vi "MultiChannelFeedbackCooling(Host).vi"(5 "RIO Device":T2="RIO0::INSTR") -> ()   [LabVIEW 2012]
doc: "This VI will will initialize the FPGA VI and then continually read and convert single point values from 4 channels of an analog input module."
uses:
  <vilib>/userdefined/High Color/nirio_resource_hc.ctl
  <vilib>/rvi/Analysis/host/Butterworth/config/Butterworth Filter Order.ctl
  <vilib>/rvi/Analysis/host/Butterworth/config/Butterworth Filter Type.ctl
  <vilib>/FPGAPlugInAG/PCIe-7841R/niLvFpga_Open_PCIe-7841R.vi
  <vilib>/FPGAPlugInAG/PCIe-7841R/niLvFpga_Run_PCIe-7841R.vi
  <vilib>/rvi/Analysis/host/Butterworth/config/BwScaledCoefficients.vi
  <vilib>/Utility/error.llb/Error Cluster From Error Code.vi
  <vilib>/rvi/errors/niLvFpgaAdjustHostInterfaceError.vi
  <vilib>/FPGAPlugInAG/PCIe-7841R/niLvFpga_Close_PCIe-7841R.vi
  <vilib>/rvi/interface/nirviOpenFPGA/nirviOpenFPGA.xnode
  MultiChannelFeed_FPGATarget2_feedbackcooling(_T5hmXv3JUos.lvbitx
  <vilib>/rvi/interface/nirviMethod/nirviMethod.xnode
  <vilib>/rvi/Analysis/host/Butterworth/XNode/ButterworthCoefficients.xnode
  <vilib>/rvi/interface/nirviReadWriteControl/nirviReadWriteControl.xnode
  <vilib>/rvi/interface/nirviCloseFPGA/nirviCloseFPGA.xnode
  <vilib>/rvi/Analysis/host/Public/NI_FpgaMspHost.lvlib
  NiFpgaLv.dll
panel:
  in  "feedback gain":fxp<+/-,32,16>
  in  "On time (s)":dbl
  in  "Off time (s)":dbl
  in  "Num cycles":u16
  in  "cycle feedback":bool
  in  "Reset after samps":u16
  in  "Num samps to reset":u16
  in  "change pars 2":bool
  in  "Delay Time (s)":dbl
  in  "Step":fxp<+/-,32,16>
  in  "End value":fxp<+/-,32,16>
  in  "ramp dc offset":bool
  in  "3, 1":fxp<+/-,32,16>
  in  "3, 2":fxp<+/-,32,16>
  in  "3, 3":fxp<+/-,32,16>=1.0
  in  "2, 3":fxp<+/-,32,16>
  in  "2, 2":fxp<+/-,32,16>=1.0
  in  "2, 1":fxp<+/-,32,16>
  in  "1, 3":fxp<+/-,32,16>
  in  "1, 2":fxp<+/-,32,16>
  in  "1,1":fxp<+/-,32,16>=1.0
  out "Feedback 2":dbl(graph)
  out "Filtered Input 2":dbl(graph)=3346.0
  out "AI2":i16(graph)=3346
  out "Feedback 1":dbl(graph)
  out "Filtered Input 1":dbl(graph)=-106.0
  out "AI1":i16(graph)=-104
  out "Feedback 0":dbl(graph)=20.0
  out "Filtered Input 0":dbl(graph)=-40.0
  out "AI0":i16(graph)=-41
  in  "Der delay 2":T1(ring)=enum."4"
  in  "Dc offset 2":fxp<+/-,32,16>
  in  "Lower lim 2":fxp<+/-,32,16>=-1000.0
  in  "Upper lim 2":fxp<+/-,32,16>=1000.0
  in  "dg 2":fxp<+/-,32,16>
  in  "pg 2":fxp<+/-,32,16>
  in  "Setpoint 2":fxp<+/-,16,16>
  in  "Der delay 1":T1(ring)=enum."4"
  in  "cutoff 1 (Hz)":dbl=50000.0
  in  "Dc offset 1":fxp<+/-,32,16>
  in  "Upper lim 1":fxp<+/-,32,16>=3600.0
  in  "Lower lim 1":fxp<+/-,32,16>=-3600.0
  in  "dg 1":fxp<+/-,32,16>
  in  "pg 1":fxp<+/-,32,16>
  in  "Setpoint 1":fxp<+/-,16,16>
  in  "sample rate (S/s)":dbl=120000.0
  in  "cutoff 0 (Hz)":dbl=50000.0
  in  "Der delay 0":T1(ring)=enum."4"
  in  "Dc offset 0":fxp<+/-,32,16>
  in  "Lower lim 0":fxp<+/-,32,16>=-3600.0
  in  "Upper lim 0":fxp<+/-,32,16>=3600.0
  in  "dg 0":fxp<+/-,32,16>=-20.0
  in  "pg 0":fxp<+/-,32,16>
  in  "Setpoint 0":fxp<+/-,16,16>
  in  "change pars":bool
  in  "stop":bool
  # "Analog Input"
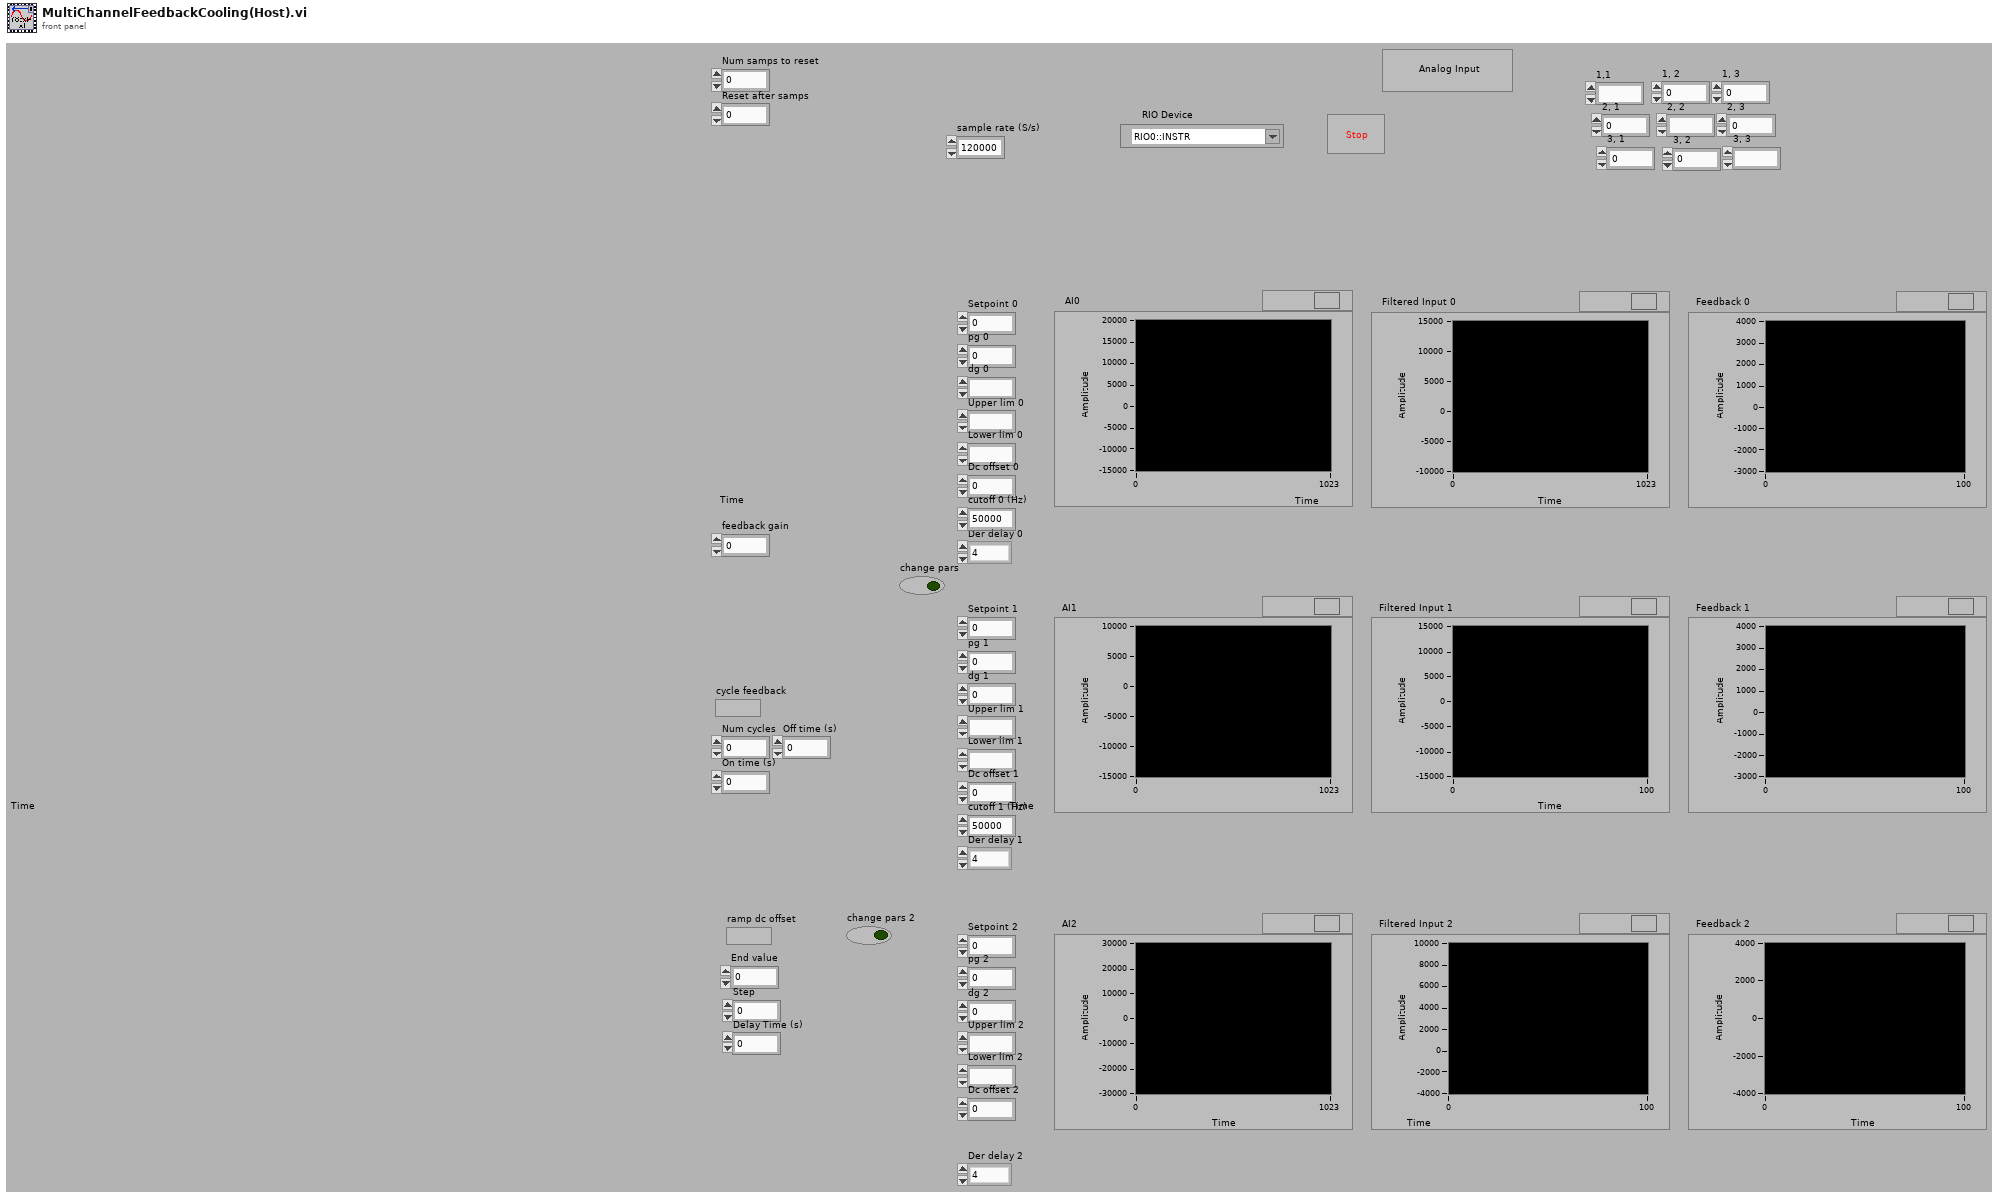
[diagram p1: front panel]
types:
  T1 = enum16{"1", "2", "4", "8", "16", "32", "64", "128", "256", "512"}
  T2 = typedef "nirio_resource_hc.ctl" = tag
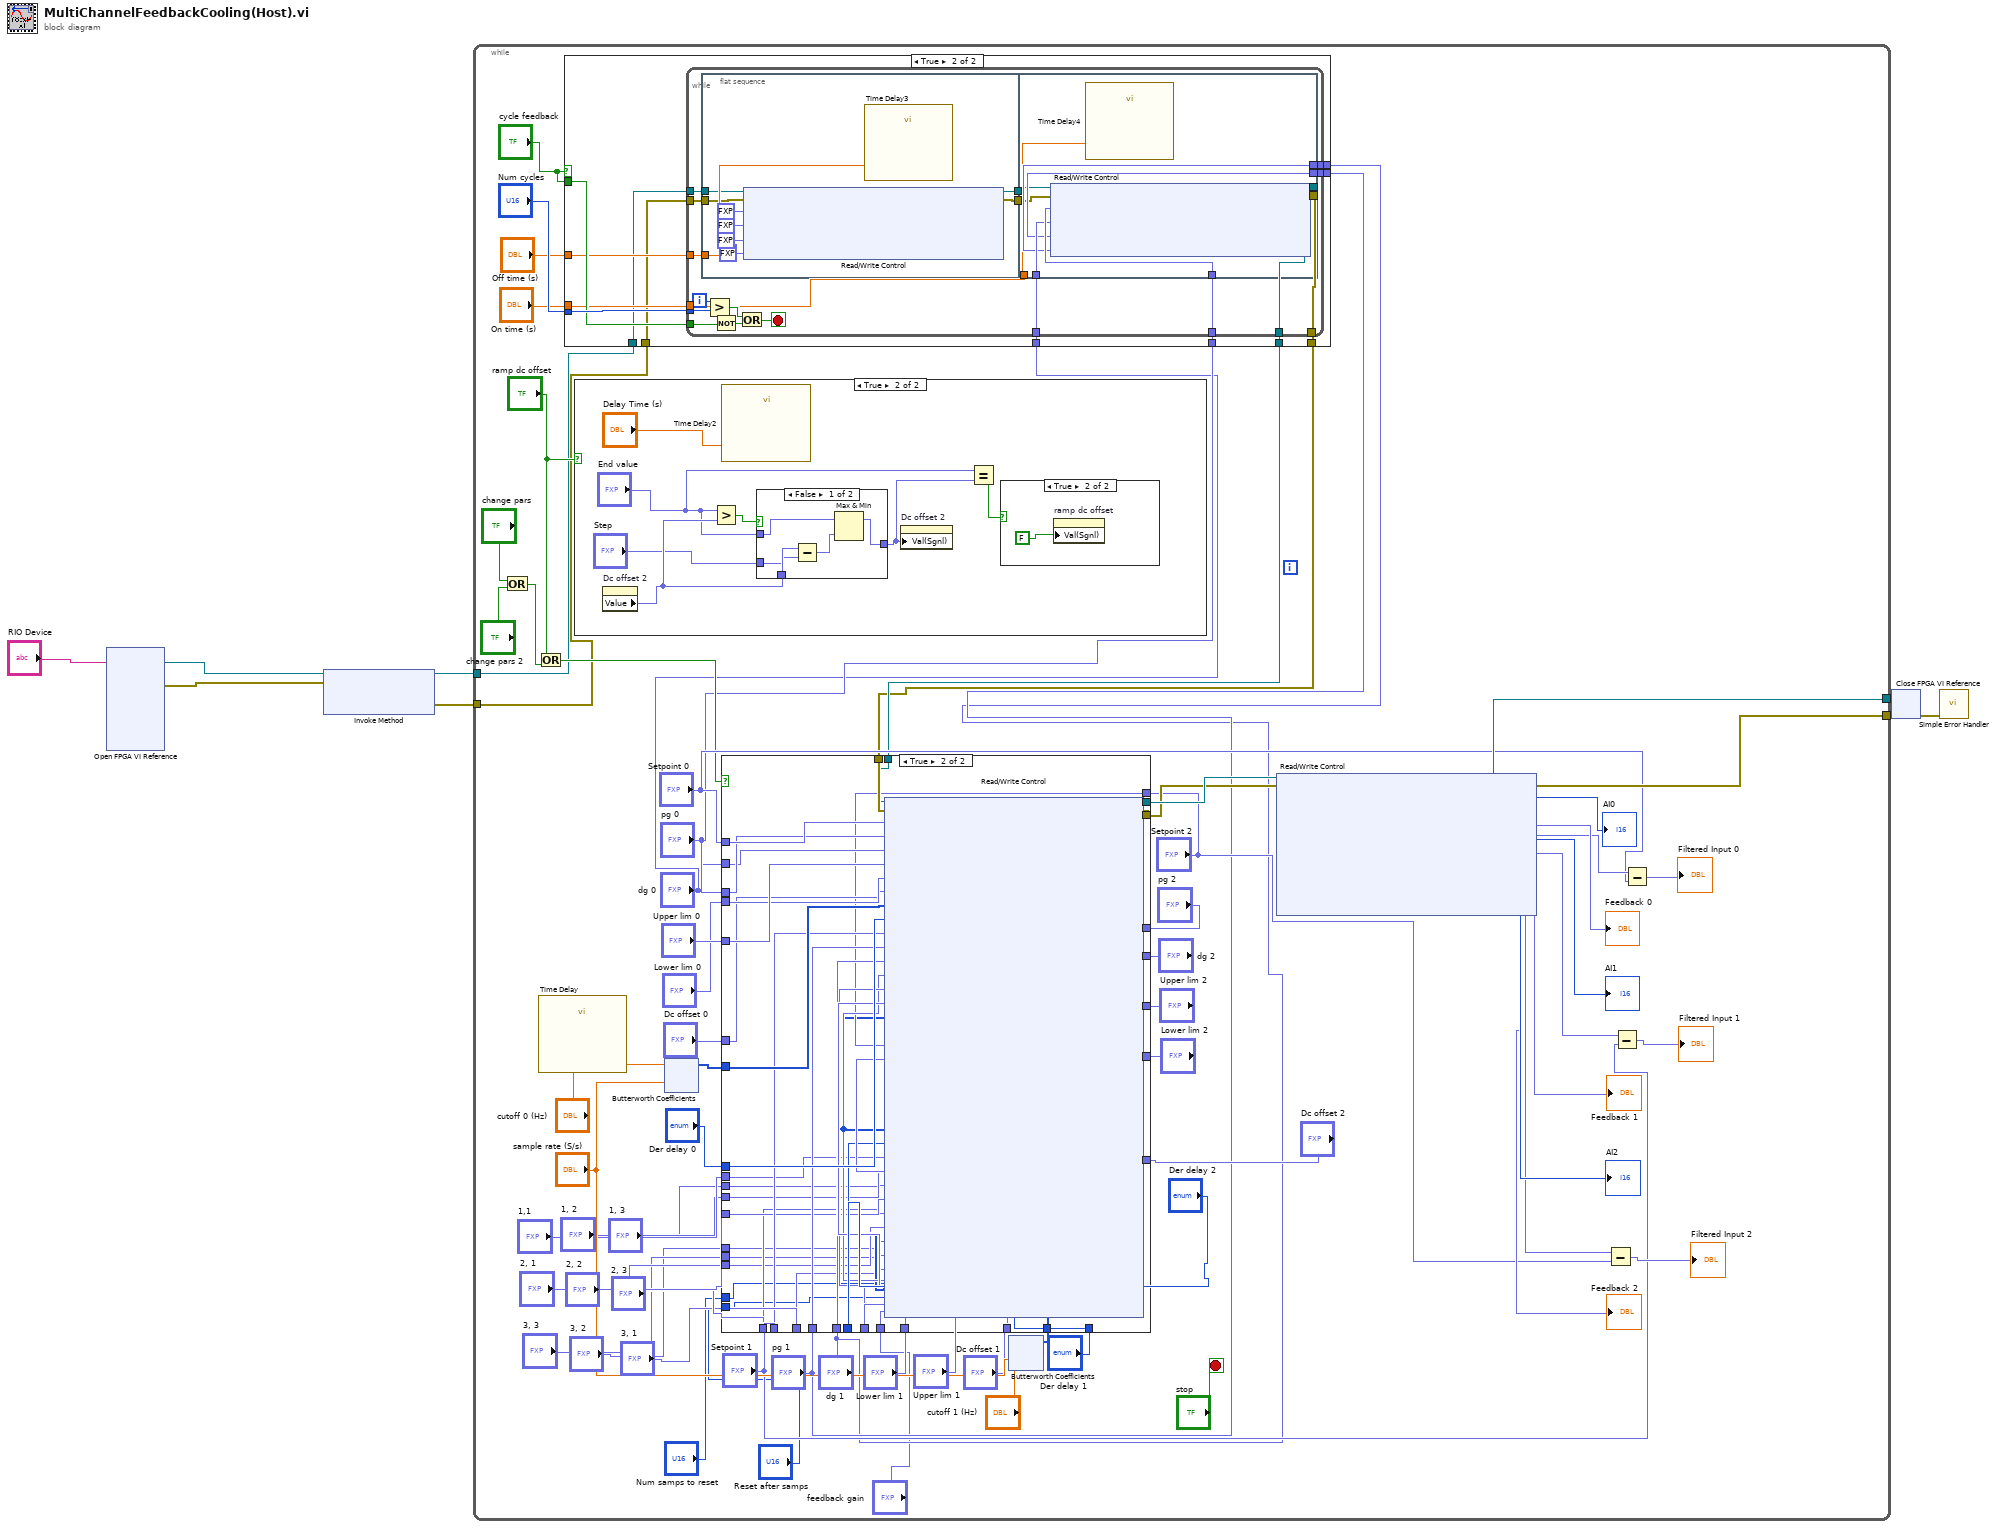
[diagram p0: block diagram]
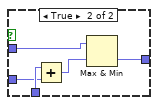
[diagram p5: hidden frame]
diagram:
  n1 = xnode "Open FPGA VI Reference"("resource name"="RIO Device") -> ("FPGA VI Reference Out"=w3:refnum<k20>, "error out"=w2:errorcluster)  [unwired: 1 in]
  n2 = xnode "Invoke Method"("FPGA VI Reference In"=w3, "error in"=w2) -> ("FPGA VI Reference Out"=w5:refnum<k20>, "error out"=w4:errorcluster)  [unwired: 1 in]
  n3 = while {
    tunnel: [w74] -> w8
    tunnel: w5 -> [w13]
    tunnel: w4 -> [w11]
    tunnel: [w73] -> w1
    stop <- "stop" stop-if-true
    n4 = Or(x="change pars", y="change pars 2") -> (x .or. y?=w24:bool)
    n5 = Or(x="ramp dc offset", y=w24) -> (x .or. y?=w27:bool)
    n6 = call "Time Delay"() -> ()  [unwired: 11 in, 1 out]
    n7 = case shown="True" "cycle feedback" {
      tunnel: "Num cycles" -> [_ w90]
      tunnel: "cycle feedback" -> [_ w89]
      tunnel: "pg 0" -> [_ w88]
      tunnel: "dg 0" -> [_ w87]
      tunnel: "pg 1" -> [_ w86]
      tunnel: "dg 1" -> [_ w85]
      tunnel: "Off time (s)" -> [_ w84]
      tunnel: "On time (s)" -> [_ w83]
      tunnel: w13 -> [w78 w82]
      tunnel: [w78 w81] -> w12
      tunnel: w11 -> [w77 w80]
      tunnel: [w77 w79] -> w10
      frame False {
      }
      frame True {
        n8 = while {
          tunnel: w90 -> [w106]
          tunnel: w89 -> [w104]
          tunnel: w88 -> [w102]
          tunnel: w87 -> [w101]
          tunnel: w86 -> [w100]
          tunnel: w85 -> [w99]
          tunnel: w84 -> [w98]
          tunnel: w83 -> [w97]
          tunnel: w82 -> [w96]
          tunnel: [w94] -> w81
          tunnel: w80 -> [w93]
          tunnel: [w91] -> w79
          i -> [w107]
          stop <- w103 stop-if-true
          n9 = flat-sequence {
            tunnel: w98 -> [w113]
            tunnel: w96 -> [w112]
            tunnel: [w111] -> w95
            tunnel: w93 -> [w110]
            tunnel: [w109] -> w92
            tunnel: w102 -> [w126]
            tunnel: w101 -> [w125]
            tunnel: w100 -> [w124]
            tunnel: w99 -> [w123]
            tunnel: w97 -> [w122]
            tunnel: w95 -> [w121]
            tunnel: [w120] -> w94
            tunnel: w92 -> [w119]
            tunnel: [w118] -> w91
            frame #0 {
              n10 = xnode "Read/Write Control"("FPGA VI Reference In"=w112, "error in"=w110, "pg 0"=fxp<+/-,32,16> 0.0, "dg 0"=fxp<+/-,32,16> 0.0, "pg 1"=fxp<+/-,32,16> 0.0, "dg 1"=fxp<+/-,32,16> 0.0) -> ("FPGA VI Reference Out"=w111:refnum<k20>, "error out"=w109:errorcluster)
              n11 = call "Time Delay3"("Delay Time (s)"=w113) -> ()  [unwired: 10 in, 1 out]
            }
            frame #1 {
              n12 = xnode "Read/Write Control"("FPGA VI Reference In"=w121, "error in"=w119, "pg 0"=w126, "dg 0"=w125, "pg 1"=w124, "dg 1"=w123) -> ("FPGA VI Reference Out"=w120:refnum<k20>, "error out"=w118:errorcluster)
              n13 = call "Time Delay4"("Delay Time (s)"=w122) -> ()  [unwired: 10 in, 1 out]
            }
          }
          n14 = Greater?(x=w107, y=w106) -> (0:w108:bool)
          n15 = Not(x=w104) -> (.not. x?=w105:bool)
          n16 = Or(x=w108, y=w105) -> (x .or. y?=w103:bool)
        }
      }
    }
    n17 = case shown="True" "ramp dc offset" {
      frame False {
      }
      frame True {
        n18 = property on="Dc offset 2" class="DigNum (strict)"() -> ("Value"=w132:fxp<+/-,32,16>)  [unwired: 2 in, 2 out]
        n19 = Greater?(x="End value", y=w132) -> (0:w133:bool)
        n20 = call "Time Delay2"("Delay Time (s)"="Delay Time (s)") -> ()  [unwired: 10 in, 1 out]
        n21 = case shown="False" w133 {
          tunnel: "End value" -> [w136 w141]
          tunnel: w132 -> [w139 w144]
          tunnel: "Step" -> [w138 w143]
          tunnel: [w135 w140] -> w131
          frame False {
            n22 = Subtract(x=w139, y=w138) -> (x-y=w137:fxp<+/-,33,17>)
            n23 = Max & Min(x=w136, y=w137) -> (max(x,y)=w135:fxp<+/-,33,17>)  [unwired: 1 out]
          }
          frame True {
            n24 = Add(x=w144, y=w143) -> (x+y=w142:fxp<+/-,33,17>)
            n25 = Max & Min(x=w141, y=w142) -> (min(x,y)=w140:fxp<+/-,33,17>)  [unwired: 1 out]
          }
        }
        n26 = property on="Dc offset 2" class="DigNum (strict)"("Val(Sgnl)"=w131) -> ()  [unwired: 2 in, 2 out]
        n27 = Equal?(x="End value", y=w131) -> (x = y?=w130:bool)
        n28 = case shown="True" w130 {
          frame False {
          }
          frame True {
            n29 = property on="ramp dc offset" class="Bool (strict)"("Val(Sgnl)"=FALSE) -> ()  [unwired: 2 in, 2 out]
          }
        }
      }
    }
    n30 = xnode "Butterworth Coefficients"("cutoff frequency (Hz)"="cutoff 0 (Hz)", "sample rate (S/s)"="sample rate (S/s)") -> ("scaled coefficients"=w68:i32[])  [unwired: 1 in, 1 out]
    n31 = xnode "Butterworth Coefficients"("cutoff frequency (Hz)"="cutoff 1 (Hz)", "sample rate (S/s)"="sample rate (S/s)") -> ("scaled coefficients"=w63:i32[])  [unwired: 1 in, 1 out]
    n32 = case shown="True" w27 {
      tunnel: w10 -> [w160 w199]
      tunnel: [w160 w198] -> w75
      tunnel: [w159 w197] -> w76
      tunnel: "Setpoint 0" -> [_ w196]
      tunnel: "pg 0" -> [_ w195]
      tunnel: "dg 0" -> [_ w194]
      tunnel: "Upper lim 0" -> [_ w193]
      tunnel: "Lower lim 0" -> [_ w192]
      tunnel: "Dc offset 0" -> [_ w191]
      tunnel: w68 -> [_ w190]
      tunnel: "Der delay 0" -> [_ w189]
      tunnel: "Der delay 1" -> [_ w188]
      tunnel: w63 -> [_ w174]
      tunnel: "Dc offset 1" -> [_ w187]
      tunnel: "Upper lim 1" -> [_ w186]
      tunnel: "Lower lim 1" -> [_ w185]
      tunnel: "dg 1" -> [_ w184]
      tunnel: "pg 1" -> [_ w183]
      tunnel: "Setpoint 1" -> [_ w182]
      tunnel: "Setpoint 2" -> [_ w181]
      tunnel: "pg 2" -> [_ w180]
      tunnel: "dg 2" -> [_ w179]
      tunnel: "Upper lim 2" -> [_ w178]
      tunnel: "Lower lim 2" -> [_ w177]
      tunnel: "Dc offset 2" -> [_ w176]
      tunnel: "Der delay 2" -> [_ w175]
      tunnel: "1,1" -> [_ w173]
      tunnel: "1, 2" -> [_ w172]
      tunnel: "1, 3" -> [_ w171]
      tunnel: "2, 1" -> [_ w170]
      tunnel: "2, 2" -> [_ w169]
      tunnel: "2, 3" -> [_ w168]
      tunnel: "3, 3" -> [_ w167]
      tunnel: "3, 2" -> [_ w166]
      tunnel: "3, 1" -> [_ w165]
      tunnel: "Num samps to reset" -> [_ w164]
      tunnel: "Reset after samps" -> [_ w163]
      tunnel: w12 -> [w159 w162]
      tunnel: "feedback gain" -> [_ w161]
      frame False {
      }
      frame True {
        n33 = xnode "Read/Write Control"("FPGA VI Reference In"=w162, "error in"=w199, "Setpoint 0"=w196, "pg 0"=w195, "dg 0"=w194, "Upper lim 0"=w193, "Lower lim 0"=w192, "Dc offset 0"=w191, "low pass coefficients 0"=w190, "Der delay 0"=w189, "Setpoint 1"=w182, "pg 1"=w183, "dg 1"=w184, "Lower lim 1"=w185, "Upper lim 1"=w186, "Dc offset 1"=w187, "low pass coefficients 1"=w174, "Der delay 1"=w188, "Setpoint 2"=w181, "pg 2"=w180, "dg 2"=w179, "Upper lim 2"=w178, "Lower lim 2"=w177, "Dc offset 2"=w176, "low pass coefficients 2"=w174, "Der de;ay 2"=w175, "1,1"=w173, "1, 2"=w172, "1, 3"=w171, "2, 1"=w170, "2, 2"=w169, "2, 3"=w168, "3, 3"=w167, "3, 2"=w166, "3, 1"=w165, "Num samps to reset"=w164, "Reset after samps"=w163, "fb gain 0"=w161) -> ("FPGA VI Reference Out"=w197:refnum<k20>, "error out"=w198:errorcluster)
      }
    }
    n34 = xnode "Read/Write Control"("FPGA VI Reference In"=w76, "error in"=w75) -> ("FPGA VI Reference Out"=w74:refnum<k20>, "error out"=w73:errorcluster, "AI0"=→"AI0":i16, "Filtered Input 0"=w41:fxp<+/-,20,20>, "Feedback 0"=→"Feedback 0":fxp<+/-,32,16>, "Connector0/AI1"=→"AI1":i16, "Filtered Input 1"=w45:fxp<+/-,20,20>, "Feedback 1"=→"Feedback 1":fxp<+/-,32,16>, "Connector0/AI2"=→"AI2":i16, "Filtered Input 2"=w48:fxp<+/-,20,20>, "Feedback 2"=→"Feedback 2":fxp<+/-,32,16>)
    n35 = Subtract(x=w48, y="Setpoint 2") -> (x-y=→"Filtered Input 2":fxp<+/-,21,21>)
    n36 = Subtract(x=w45, y="Setpoint 1") -> (x-y=→"Filtered Input 1":fxp<+/-,21,21>)
    n37 = Subtract(x=w41, y="Setpoint 0") -> (x-y=→"Filtered Input 0":fxp<+/-,21,21>)
  }
  n38 = xnode "Close FPGA VI Reference"("FPGA VI Reference In"=w8, "error in"=w1) -> ("error out"=w7:errorcluster)
  n39 = call <vilib>:"Simple Error Handler.vi"("error in (no error)"=w7) -> ()  [unwired: 4 in, 5 out]
